vi "GetSerializationDetails.vi"(8 "error in (no error)":errorcluster, 11 "FileConverterBase in":refnum<class "FileConverterBase.lvclass">) -> (0 "error out":errorcluster, 1 "ID":string, 2 "FileType":T1, 3 "FileConverterBase out":refnum<class "FileConverterBase.lvclass">, 4 "ComponentsSerialized":string)   [LabVIEW 2017, in "FileConverterBase.lvclass"]
uses:
  FileConverterBase.lvclass
  SupportedFileTypes.ctl
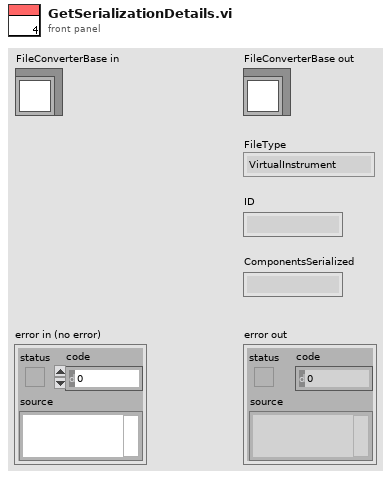
[diagram p1: front panel]
types:
  T1 = typedef "SupportedFileTypes.ctl" = enum16{"VirtualInstrument", "Polymorphic VI", "Class", "Project"}
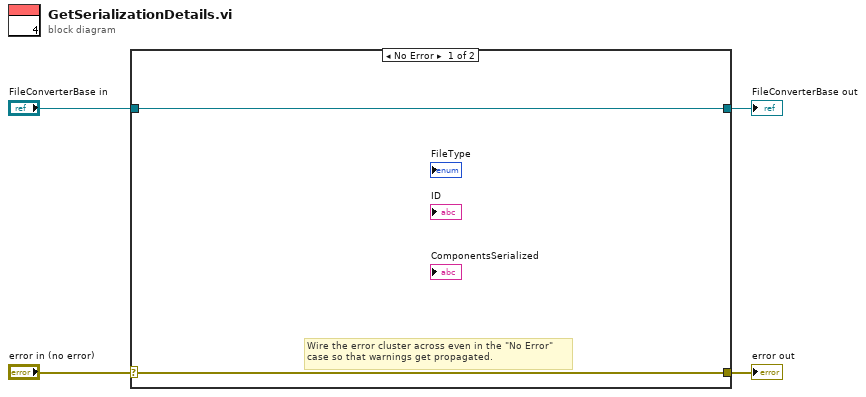
[diagram p0: block diagram]
diagram:
  n1 = case shown="No Error" "error in (no error)" {
    selector: "error in (no error)" -> [w5 w8]
    tunnel: [w5 w8] -> w3
    tunnel: [w6 w7] -> w1
    tunnel: "FileConverterBase in" -> [w6 w7]
    frame No Error {
      # "Wire the error cluster across even in the \"No Error\"\ncase so that warnings get propagated."
    }
    frame Error {
    }
  }
  "error out" <- w3
  "FileConverterBase out" <- w1
